vi "Draw Mine Array.vi"(8 "Error In":errorcluster, 10 "Box Array":cluster{"x":i16, "y":i16}[](array[cluster]), 11 "Picture In":picture) -> (0 "Error Out":errorcluster, 3 "Picture Out":picture)   [LabVIEW 2011]
doc: "Places an icon of a mine at the indexes specified by Mine Index Array, each a 50px by 50px box."
uses:
  <vilib>/picture/picture.llb/Draw 8-Bit Pixmap.vi
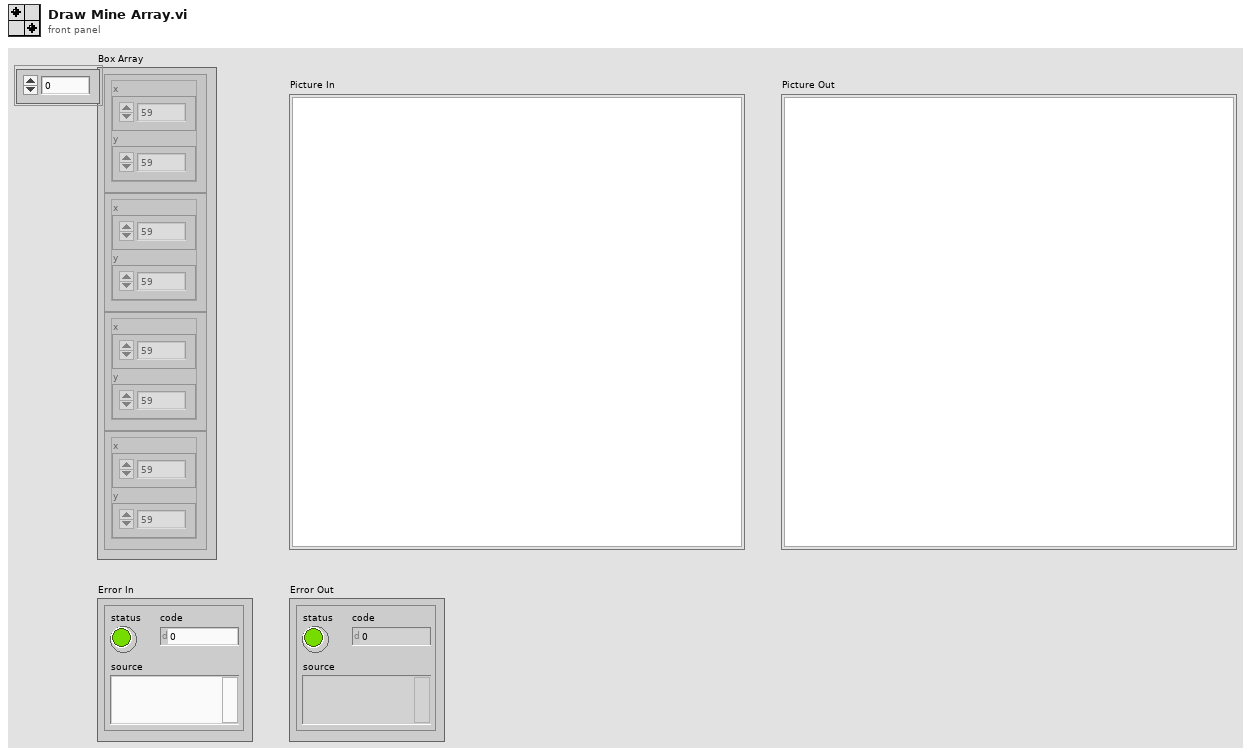
[diagram p1: front panel]
types:
  T1 = typedef "imagedata.ctl" = cluster{"image type":i32, "image depth":i32, "image":u8[], "mask":u8[], "colors":u32[], "Rectangle":cluster{"left":i16, "top":i16, "right":i16, "bottom":i16}}
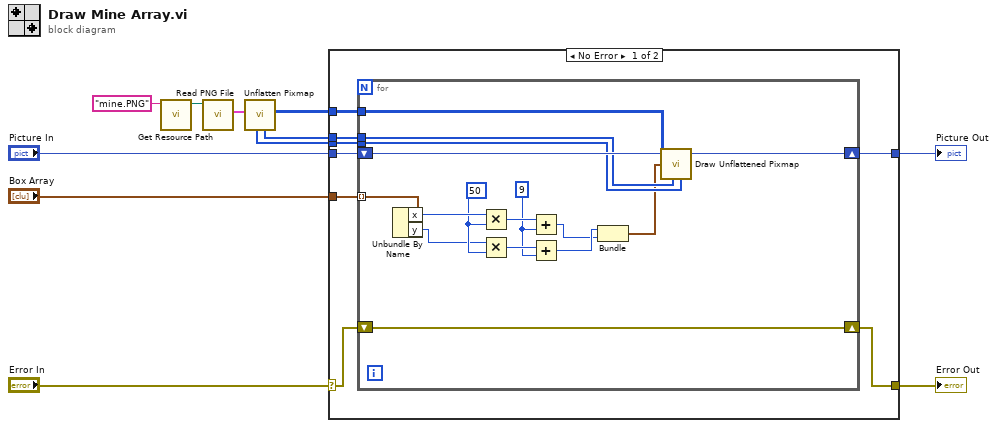
[diagram p0: block diagram]
diagram:
  n1 = call "Get Resource Path.vi"("Resource Filename"="mine.PNG" ("resource filename")) -> ("Resource Path"=w4:path)  [unwired: 9 in, 1 out]
  n2 = call <vilib>:"Read PNG File.vi"("path to PNG file"=w4) -> ("image data"=w11:T1)  [unwired: 8 in, 2 out]
  n3 = call <vilib>:"Unflatten Pixmap.vi"("image data"=w11) -> ("8-bit pixmap"=w9:u8[][], "colors"=w6:u32[], "mask"=w7:u8[])  [unwired: 4 in, 4 out]
  n4 = case shown="No Error" "Error In" {
    selector: "Error In" -> [w12 w36]
    tunnel: "Box Array" -> [w19 _]
    tunnel: w9 -> [w18 _]
    tunnel: [w17 w37] -> w8
    tunnel: w7 -> [w16 _]
    tunnel: w6 -> [w15 _]
    tunnel: "Picture In" -> [w14 w37]
    tunnel: [w13 w36] -> w1
    frame No Error {
      n5 = for {
        tunnel: w19 -> [w34] mode=indexing
        tunnel: w18 -> [w35]
        shift-right: [w27] -> w17
        shift-left: w14 -> [w26]
        tunnel: w16 -> [w24]
        tunnel: w15 -> [w25]
        shift-right: [w20] -> w13
        shift-left: w12 -> [w20]
        w28 = i16 9
        w32 = i16 50
        n6 = Unbundle By Name(w34) -> ("x"=w33:i16, "y"=w31:i16)
        n7 = Multiply(x=w33, y=w32) -> (x*y=w30:i16)
        n8 = Multiply(x=w31, y=w32) -> (x*y=w29:i16)
        n9 = Add(x=w30, y=w28) -> (x+y=w21:i16)
        n10 = Add(x=w29, y=w28) -> (x+y=w22:i16)
        n11 = Bundle(w22, w21) -> (w23:cluster{i16, i16})  [unwired: 1 in]
        n12 = call-poly <vilib>:"Draw Unflattened Pixmap.vi"("picture"=w26, "top left point(0, 0)"=w23, "data"=w35, "color table"=w25, "mask"=w24) -> ("new picture"=w27:picture)  [unwired: 4 in]
      }
    }
    frame Error {
    }
  }
  "Picture Out" <- w8
  "Error Out" <- w1
